vi "Write Directors.vi"(8 "error in (no error)":errorcluster, 10 "Directors":refnum<class "CommandDirector.lvclass">[](array[class]), 11 "InteractionProcessor in":refnum<class "InteractionProcessor.lvclass">) -> (0 "error out":errorcluster, 3 "InteractionProcessor out":refnum<class "InteractionProcessor.lvclass">)   [LabVIEW 2023, in "HAF.lvlib" / "InteractionProcessor.lvclass"]
doc: "Sets a new collection of CommandDirectors."
uses:
  InteractionProcessor.lvclass
  CommandDirector/CommandDirector.lvclass
  InteractionProcessor.lvclass/InteractionProcessor.ctl
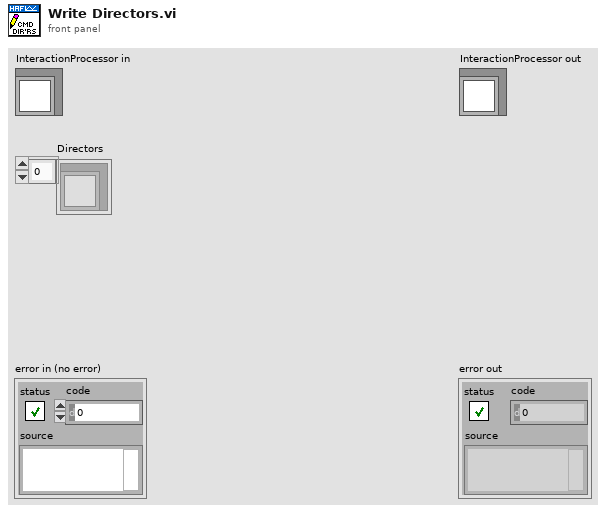
[diagram p1: front panel]
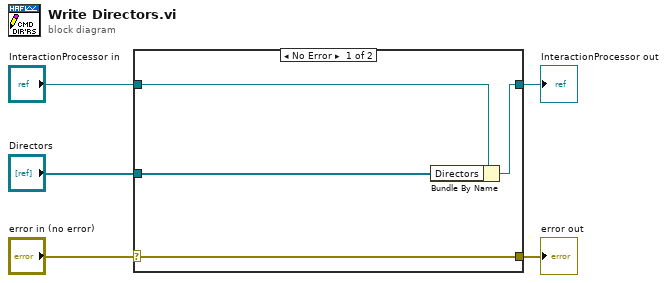
[diagram p0: block diagram]
diagram:
  n1 = case shown="No Error" "error in (no error)" {
    selector: "error in (no error)" -> [w9 w10]
    tunnel: [w9 w10] -> w4
    tunnel: [w7 w11] -> w2
    tunnel: "InteractionProcessor in" -> [w8 w11]
    tunnel: "Directors" -> [w6 _]
    frame No Error {
      n2 = Bundle By Name(cluster=w8, "Directors"=w6) -> (w7:refnum<class "InteractionProcessor.lvclass">)
    }
    frame Error {
    }
  }
  "error out" <- w4
  "InteractionProcessor out" <- w2
